vi "Base 64.vi"() -> ()   [LabVIEW 2017]
uses:
  <vilib>/LabVIEW Open Source Project/OpenSerializer.Base64/Base64_ByteLUT.vi
  <vilib>/LabVIEW Open Source Project/OpenSerializer.Base64/Base64_CharSet.vi
  <vilib>/LabVIEW Open Source Project/OpenSerializer.Base64/Serializer.Base64.lvclass
panel:
  in  "Base64 String":string
  out "Encoded String":string
  out "Decoded String":string
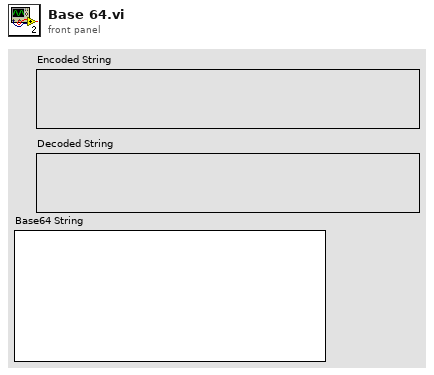
[diagram p1: front panel]
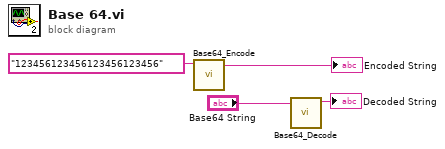
[diagram p0: block diagram]
diagram:
  n1 = call <vilib>:"Base64_Encode.vi"("String"="123456123456123456123456") -> ("Encoded String"=→"Encoded String":string)  [unwired: 9 in, 1 out]
  n2 = call <vilib>:"Base64_Decode.vi"("Base64 String"="Base64 String") -> ("Decoded String"=→"Decoded String":string)  [unwired: 9 in, 1 out]
